vi "calculate Z CUDA.vi"(6 "拟合半径":i32=2, 7 "info":T3[](array[typedef]), 8 "y_qi":sgl[][](array[numeric]), 9 "x_qi":sgl[][](array[numeric]), 10 "beads track":T1[](array[typedef]) {"centroid"."Y Centroid" format="%.2f"; "centroid"."X Centroid" format="%.2f"; "ROI Des out"."Contours"."Type" items=["No Selection", "Point", "Line", "Rectangle", "Oval", "Polygon", "Freehand Region", "Annulus", "Unused2", "Unused3", "Broken Line", "Freehand Line", "Rotated Rectangle"]}) -> (2 "tracking out":T1[](array[typedef]) {"centroid"."Y Centroid" format="%.2f"; "centroid"."X Centroid" format="%.2f"; "ROI Des out"."Contours"."Type" items=["No Selection", "Point", "Line", "Rectangle", "Oval", "Polygon", "Freehand Region", "Annulus", "Unused2", "Unused3", "Broken Line", "Freehand Line", "Rotated Rectangle"]}, 3 "Dif LUT":cluster{"LUT":dbl[], dbl[]}[](graph))   [LabVIEW 2017]
uses:
  control/bead info.ctl
  <vilib>/vision/Image Controls.llb/IMAQ Image.ctl
  control/Bead track.ctl
  <vilib>/Analysis/NI_AALPro.lvlib
panel:
  out "xyz value":dbl[][](array[numeric])
  out "min LUT":cluster{dbl[], "Best Polynomial Fit":dbl[]}(graph)
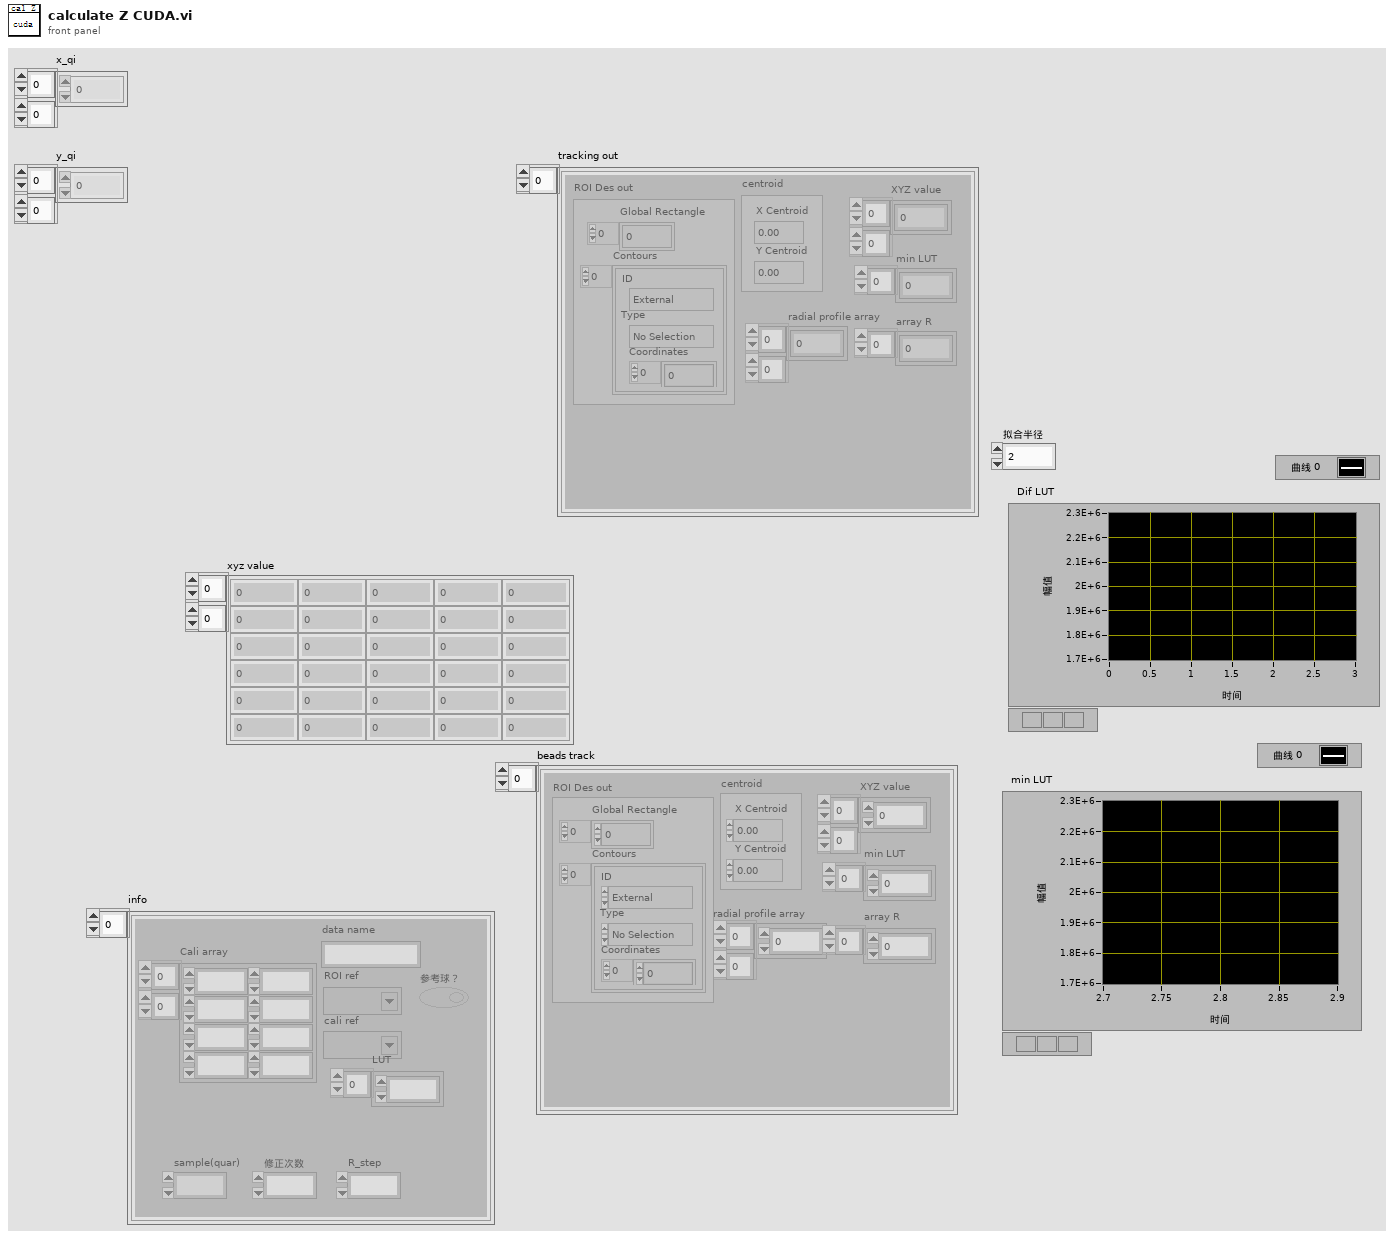
[diagram p1: front panel]
types:
  T1 = typedef "Bead track.ctl" = cluster{"XYZ value":dbl[][], "radial profile array":dbl[][], "min LUT":dbl[], "ROI Des out":T2, "array R":dbl[], "centroid":cluster{"X Centroid":sgl, "Y Centroid":sgl}}
  T2 = typedef "ROI Descriptor" = cluster{"Global Rectangle":i32[], "Contours":cluster{"ID":enum32{"External", "Internal"}, "Type":u32, "Coordinates":i32[]}[]}
  T3 = typedef "bead info.ctl" = cluster{"data name":string, "ROI ref":T4, "cali ref":T4, "参考球？":bool, "LUT":dbl[], "Cali array":dbl[][], "修正次数":i32, "R_step":dbl, "sample(quar)":i32}
  T4 = typedef "IMAQ Image.ctl" = refnum<image>
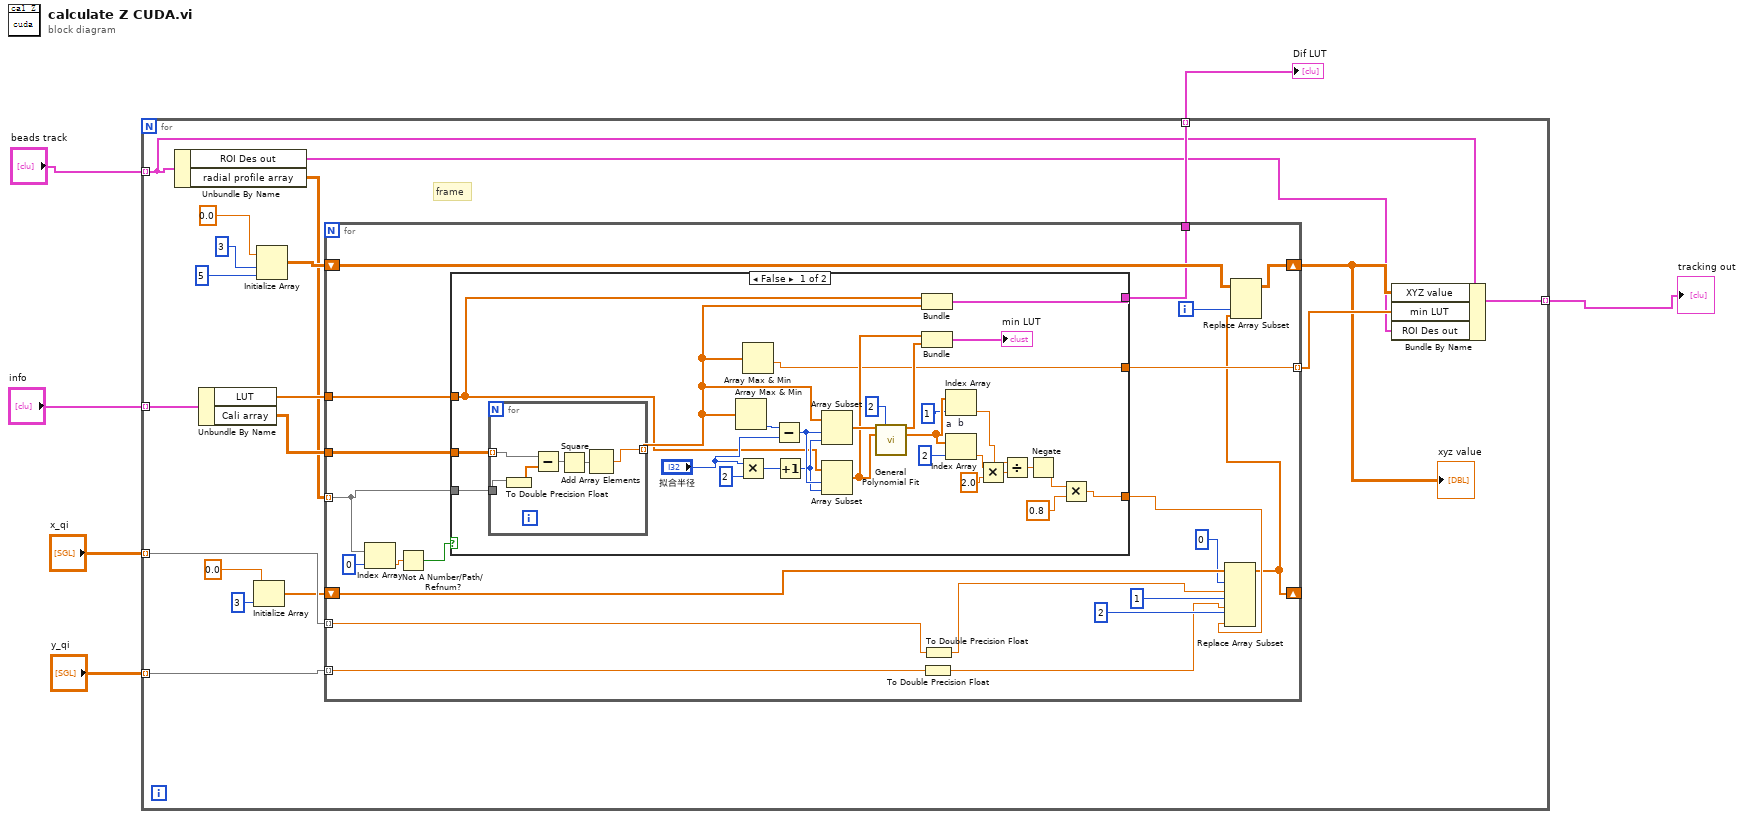
[diagram p0: block diagram]
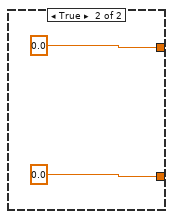
[diagram p2: hidden frame]
diagram:
  n1 = for {
    tunnel: "beads track" -> [w10] mode=indexing
    tunnel: "info" -> [w17] mode=indexing
    tunnel: [w16] -> w5 mode=indexing
    tunnel: [w15] -> w4 mode=indexing
    tunnel: "x_qi" -> [w12] mode=indexing
    tunnel: "y_qi" -> [w11] mode=indexing
    # "frame"
    n2 = Unbundle By Name(w10) -> ("ROI Des out"=w14:T2, "radial profile array"=w13:dbl[][])
    n3 = Unbundle By Name(w17) -> ("LUT"=w21:dbl[], "Cali array"=w20:dbl[][])
    n4 = Initialize Array(0.0 ("element"), 3 ("dimension size")) -> (w7:dbl[])
    n5 = Initialize Array(0.0 ("元素"), 3 ("维数大小"), 5 ("dimension size")) -> (w25:dbl[][])
    n6 = for "For循环" {
      tunnel: w13 -> [w40] mode=indexing
      shift-right: [w45] -> w18
      shift-left: w25 -> [w46]
      tunnel: [w44] -> w23 mode=indexing
      tunnel: w21 -> [w43]
      tunnel: w20 -> [w42]
      tunnel: [w36] -> w15
      tunnel: w12 -> [w35] mode=indexing
      tunnel: w11 -> [w34] mode=indexing
      shift-right: [w26] -> _
      shift-left: w7 -> [w33]
      i -> [w41]
      n7 = Index Array(array=w40, index=0 ("索引")) -> (element=w38:dbl)
      n8 = Not A Number/Path/Refnum?(number/path/refnum=w38) -> (NaN/Path/Refnum?=w37:bool)
      n9 = case shown="False" w37 {
        tunnel: [w53 0.0] -> w27
        tunnel: [w51 0.0] -> w44
        tunnel: w43 -> [w50 _]
        tunnel: w42 -> [w49 _]
        tunnel: w40 -> [w48 _]
        tunnel: [w47 _] -> w36
        frame False {
          n10 = for "For循环" {
            tunnel: w48 -> [w80]
            tunnel: [w77] -> w52 mode=indexing
            tunnel: w49 -> [w76] mode=indexing
            n11 = To Double Precision Float(number=w80) -> (double precision float=w75:dbl[])
            n12 = Subtract(x=w76, y=w75) -> (x-y=w79:dbl[])
            n13 = Square(x=w79) -> (x^2=w78:dbl[])
            n14 = Add Array Elements(numeric array=w78) -> (sum=w77:dbl)
          }
          n15 = Array Max & Min(array=w52) -> (min index (indices)=w60:i32)  [unwired: 3 out]
          n16 = Multiply(x="拟合半径", y=2 ("x")) -> (x*y=w64:i32)
          n17 = Array Max & Min(array=w52) -> (min value=w51:dbl)  [unwired: 3 out]
          n18 = Subtract(x=w60, y="拟合半径") -> (x-y=w62:i32)
          n19 = Increment(x=w64) -> (x+1=w61:i32)
          n20 = Array Subset(array=w52, index=w62, length=w61) -> (w59:dbl[])
          n21 = Array Subset(array=w50, index=w62, length=w61) -> (w57:dbl[])
          n22 = call <vilib>:"General Polynomial Fit.vi"("Y"=w59, "polynomial order"=2, "X"=w57) -> ("Best Polynomial Fit"=w58:dbl[], "Polynomial Coefficients"=w72:dbl[])  [unwired: 9 in, 2 out]
          n23 = Bundle("LUT"=w50, w52) -> (w47:cluster{"LUT":dbl[], dbl[]})  [unwired: 1 in]
          n24 = Bundle(w57, "Best Polynomial Fit"=w58) -> (→"min LUT":cluster{dbl[], "Best Polynomial Fit":dbl[]})  [unwired: 1 in]
          n25 = Index Array "b"(array=w72, index=1 ("索引")) -> (element=w68:dbl)
          n26 = Index Array "a"(array=w72, index=2 ("索引")) -> (element=w70:dbl)
          n27 = Multiply(x=w70, y=2.0) -> (x*y=w67:dbl)
          n28 = Divide(x=w68, y=w67) -> (x/y=w66:dbl)
          n29 = Negate(x=w66) -> (-x=w55:dbl)
          n30 = Multiply(x=w55, y=0.8) -> (x*y=w53:dbl)
        }
        frame True {
        }
      }
      n31 = To Double Precision Float(number=w34) -> (double precision float=w28:dbl)
      n32 = To Double Precision Float(number=w35) -> (double precision float=w29:dbl)
      n33 = Replace Array Subset(array=w33, new element #1=w29, index #1=0 ("index"), new element #2=w28, index #2=1 ("index"), new element #3=w27, index #3=2 ("index")) -> (w26:dbl[])
      n34 = Replace Array Subset(array=w46, new element=w26, index (col)=w41) -> (w45:dbl[][])  [unwired: 1 in]
    }
    "xyz value" <- w18
    n35 = Bundle By Name(cluster=w10, "XYZ value"=w18, "min LUT"=w23, "ROI Des out"=w14) -> (w16:T1)
  }
  "tracking out" <- w5
  "Dif LUT" <- w4
